vi "simple acq - used for Insight.vi"() -> ()   [LabVIEW 2015]
uses:
  AlazarTech/ATS-VI/6.0.8/ATS_ctl/ATS_Async_Status.ctl
  AlazarTech/ATS-VI/6.0.8/ATS_ctl/ATS_Global.ctl
  AlazarTech/ATS-VI/6.0.8/ATS_ctl/Record.ctl
  AlazarTech/ATS-VI/6.0.8/ATS_ctl/Clock.ctl
  AlazarTech/ATS-VI/6.0.8/ATS_ctl/ClockSource.ctl
  AlazarTech/ATS-VI/6.0.8/ATS_ctl/ClockRate.ctl
  AlazarTech/ATS-VI/6.0.8/ATS_ctl/ClockEdge.ctl
  AlazarTech/ATS-VI/6.0.8/ATS_ctl/InputCtrl.ctl
  AlazarTech/ATS-VI/6.0.8/ATS_ctl/Coupling.ctl
  AlazarTech/ATS-VI/6.0.8/ATS_ctl/Range.ctl
  AlazarTech/ATS-VI/6.0.8/ATS_ctl/Impedance.ctl
  AlazarTech/ATS-VI/6.0.8/ATS_ctl/Bandwidth.ctl
  AlazarTech/ATS-VI/6.0.8/ATS_ctl/Trigger.ctl
  AlazarTech/ATS-VI/6.0.8/ATS_ctl/TriggerOperation.ctl
  AlazarTech/ATS-VI/6.0.8/ATS_ctl/TriggerEngine.ctl
  AlazarTech/ATS-VI/6.0.8/ATS_ctl/ExtTrigger.ctl
  AlazarTech/ATS-VI/6.0.8/ATS_ctl/ExtTrigRange.ctl
  AlazarTech/ATS-VI/6.0.8/ATS_ctl/ATS_Async_Ctrl.ctl
  AlazarTech/ATS-VI/6.0.8/ATS_ctl/ATS_Async_Mode.ctl
  AlazarTech/ATS-VI/6.0.8/ATS_ctl/ATS_Async_Setting.ctl
  AlazarTech/ATS-VI/6.0.8/ATS_ctl/ATS_DMA_Channel.ctl
  AlazarTech/ATS-VI/6.0.8/ATS_ctl/ATS_ReadSamples.ctl
  AlazarTech/ATS-VI/6.0.8/ATS_ctl/Device_Ctrl.ctl
  <vilib>/Utility/file.llb/Read From Spreadsheet File (DBL).vi
panel:
  in  "saving":bool
  out "Record.Length":u32
  out "offset":i16
  out "mult":dbl
  in  "result":bool
  out "path":path
  in  "save sweep":bool
  in  "use DVV":bool=TRUE
  out "dvv":dbl[](array[numeric]) format="%0.3f"
  in  "file path (dialog if empty)":path=path "\\\\192.168.1.100\\data/DVV.txt"
  in  "Setup_In":T1={"Record"={"Count"=1, "Presize"=0, "Length"=2784}, "Clock"={"ClckSource"=enum."External", "ClckRate"=12, "ClckEdge"=0, "Decimation"=0}, "Input A"={"Coupling"=enum."DC", "Range"=5, "Impedance"=enum."50 ohms", "Bandwidth"=enum."Full Bandwidth"}, "Input B"={"Coupling"=enum."DC", "Range"=6, "Impedance"=enum."50 ohms", "Bandwidth"=enum."Full Bandwidth"}, "Trigger"={"TrigOperation"=enum."Only X", "Timeout (s)"=1.0, "Trig. Delay"=0, "Engine X"={"Source"=enum."External", "Slope"=enum."Positive", "Level"=150}, "Engine Y"={"Source"=enum."Disable", "Slope"=enum."Positive", "Level"=128}, "ExtTrigControl"={"Coupling"=enum."DC", "Range"=enum."TTL"}}} {"Clock"."ClckEdge" items=["Rising", "Falling"]; "Clock"."ClckRate" items=["1 kS/s", "2 kS/s", "5 kS/s", "10 kS/s", "20 kS/s", "50 kS/s", "100 kS/s", "200 kS/s", "500 kS/s", "1 MS/s", "2 MS/s", "5 MS/s", "10 MS/s", "20 MS/s", "50 MS/s", "100 MS/s", "250 MS/s", "500 MS/s"]; "Input B"."Range" items=["40mV", "100mV", "200mV", "400mV", "1 V", "2 V", "4 V"]; "Trigger"."Timeout (s)" format="%.2f"; "Input A"."Range" items=["40mV", "100mV", "200mV", "400mV", "1 V", "2 V", "4 V"]}
  out "Async_Status":T17
  out "error out":errorcluster
  out "Waveform Graph":dbl[](graph)
  in  "Stop Button":bool
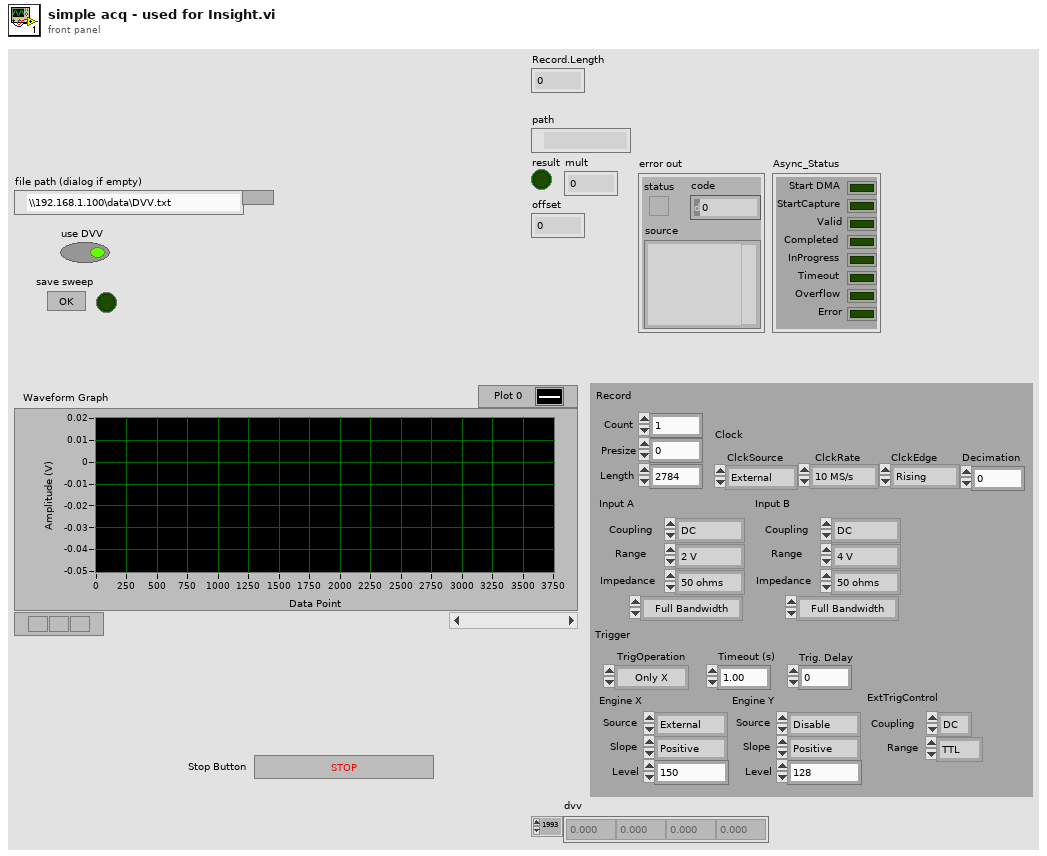
[diagram p1: front panel]
types:
  T1 = typedef "ATS_Global.ctl" = cluster{"Record":T2, "Clock":T3, "Input A":T7, "Input B":T7, "Trigger":T12}
  T2 = typedef "Record.ctl" = cluster{"Count":u32, "Presize":u32, "Length":u32}
  T3 = typedef "Clock.ctl" = cluster{"ClckSource":T4, "ClckRate":T5, "ClckEdge":T6, "Decimation":u32}
  T4 = typedef "ClockSource.ctl" = enum16{"Internal", "External", "Medium Ext.", "Slow Ext.", "Ext. AC", "Ext. DC", "Ext. (PLL)"}
  T5 = typedef "ClockRate.ctl" = u32
  T6 = typedef "ClockEdge.ctl" = u16
  T7 = typedef "InputCtrl.ctl" = cluster{"Coupling":T8, "Range":T9, "Impedance":T10, "Bandwidth":T11}
  T8 = typedef "Coupling.ctl" = enum16{"AC", "DC"}
  T9 = typedef "Range.ctl" = u32
  T10 = typedef "Impedance.ctl" = enum16{"1M ohms", "50 ohms"}
  T11 = typedef "Bandwidth.ctl" = enum16{"Full Bandwidth", "Reduce Bandwidth"}
  T12 = typedef "Trigger.ctl" = cluster{"TrigOperation":T13, "Timeout (s)":dbl, "Trig. Delay":u32, "Engine X":T14, "Engine Y":T14, "ExtTrigControl":T15}
  T13 = typedef "TriggerOperation.ctl" = enum16{"Only X", "Only Y", "X or Y", "X and Y", "X xor Y", "X and not Y", "not X and Y"}
  T14 = typedef "TriggerEngine.ctl" = cluster{"Source":enum32{"Chan_A", "Chan_B", "External", "Disable"}, "Slope":enum32{"Positive", "Negative"}, "Level":u32}
  T15 = typedef "ExtTrigger.ctl" = cluster{"Coupling":T8, "Range":T16}
  T16 = typedef "ExtTrigRange.ctl" = enum16{"1 V", "5 V", "TTL"}
  T17 = typedef "ATS_Async_Status.ctl" = cluster{"Start DMA":bool, "StartCapture":bool, "Valid":bool, "Completed":bool, "InProgress":bool, "Timeout":bool, "Overflow":bool, "Error":bool}
  T18 = typedef "ATS_ReadSamples.ctl" = cluster{"Offset":i32, "Length":u32}
  T19 = typedef "ATS_DMA_Channel.ctl" = enum16{"Channel_A", "Channel_B", "A & B"}
  T20 = typedef "ATS_Async_Setting.ctl" = cluster{"UseHeader":u32, "Rec/Buffer":u32, "Total_Rec":u32, "DataBuffer":bool, "GetProcessedData":bool}
  T21 = typedef "ATS_Async_Mode.ctl" = enum16{"Continuous", "Triggered", "No-Pre-Trigger", "Traditional"}
  T22 = typedef "ATS_Async_Ctrl.ctl" = enum16{"SetupDMA", "StartCapture", "Get", "Get_Stream", "Abort", "Stop"}
  T23 = typedef "Device_Ctrl.ctl" = enum16{"Status", "About", "Arm", "ForceTrig", "Abort", "Initialize", "Init (NoPreset)", "Info", "Close", "Calibrate", "SetManually", "LED_ON", "LED_OFF"}
  T24 = enum16{"open", "replace", "create", "open or create", "replace or create", "replace or create with confirmation"}
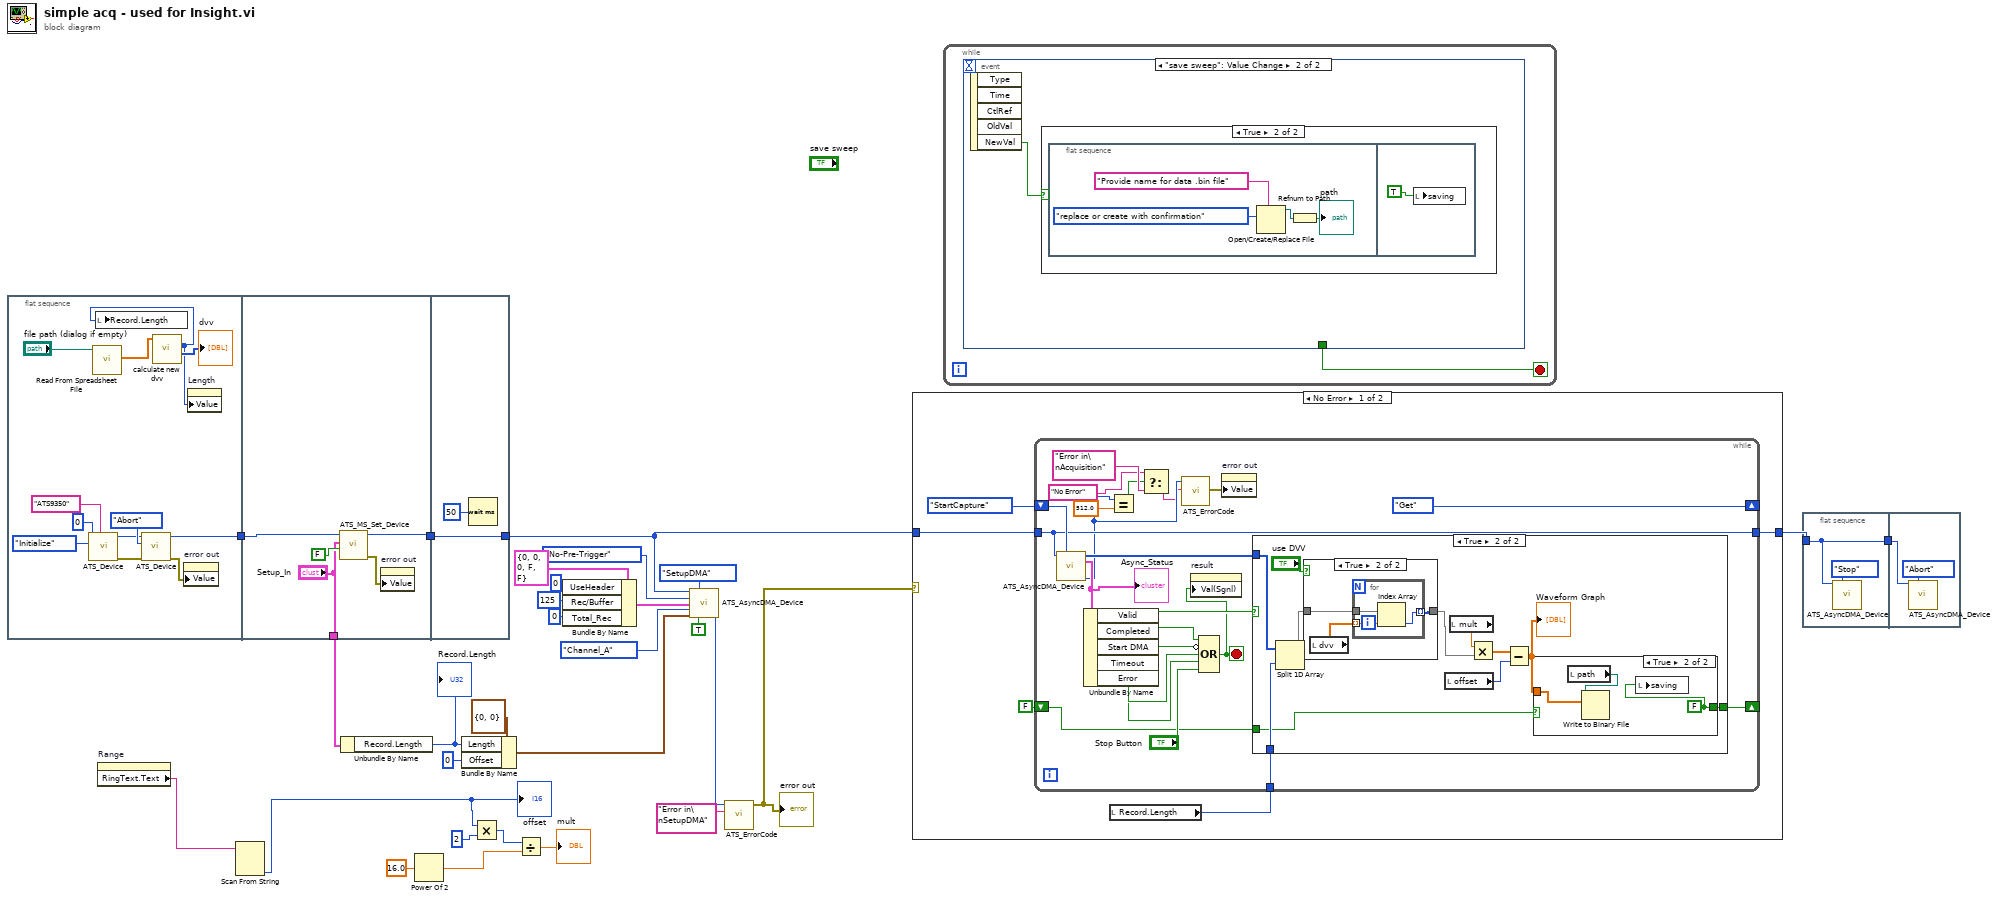
[diagram p0: block diagram]
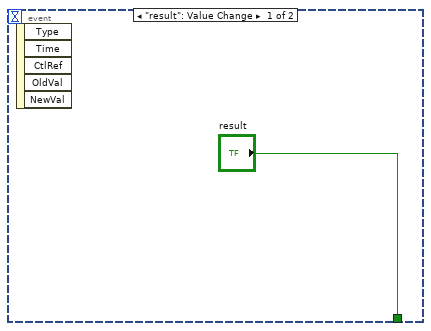
[diagram p2: hidden frame]
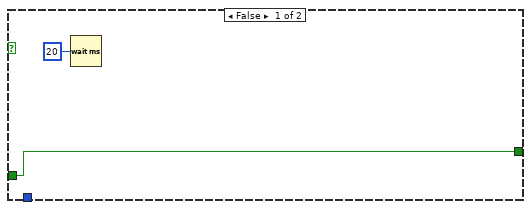
[diagram p4: hidden frame]
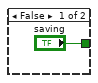
[diagram p5: hidden frame]
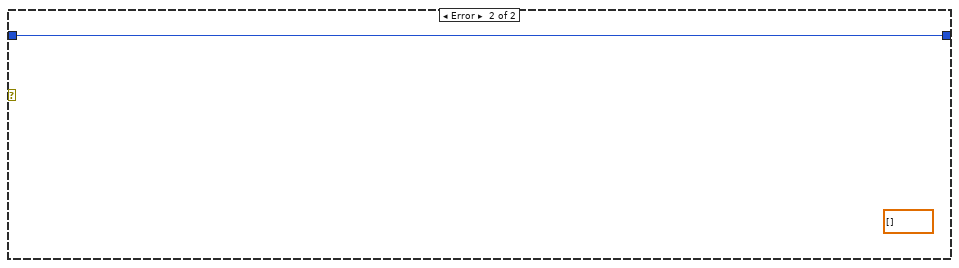
[diagram p7: hidden frame]
diagram:
  n1 = flat-sequence {
    tunnel: [w35] -> w26
    tunnel: w26 -> [w46]
    tunnel: [w45] -> w25
    tunnel: ["Setup_In"] -> w8
    tunnel: [w47] -> w27
    tunnel: w25 -> [w47]
    frame #0 {
      n2 = call "ATS_Device.vi"("BoardToVerify"="ATS9350", "DevCtrl"=Device_Ctrl."Initialize", "DeviceIn"=0 ("Device")) -> ("error out"=w40:errorcluster, "DeviceOut"=w36:i32)  [unwired: 2 in, 5 out]
      n3 = call-poly <vilib>:"Read From Spreadsheet File.vi"("file path (dialog if empty)"="file path (dialog if empty)") -> ("first row"=w32:dbl[])  [unwired: 6 in, 4 out]
      n4 = call "ATS_Device.vi"("error in (no error)"=w40, "DevCtrl"=Device_Ctrl."Abort", "DeviceIn"=w36) -> ("error out"=w34:errorcluster, "DeviceOut"=w35:i32)  [unwired: 2 in, 5 out]
      n5 = call "calculate new dvv.vi"("dvv"=w32) -> ("DVV*"=→"dvv":u32[], "Record Points"=w30:i32)  [unwired: 9 in]
      n6 = local write "Record.Length"(w30) -> ()
      n7 = property on="error out" class="Clust (strict)"("Value"=w34) -> ()  [unwired: 2 in, 2 out]
      n8 = property on="Length" class="DigNum (strict)"("Value"=w30) -> ()  [unwired: 2 in, 2 out]
    }
    frame #1 {
      n9 = call "ATS_MS_Set_Device.vi"("Set_Manually (F)"=FALSE, "Setup_In"="Setup_In", "DeviceIn"=w46) -> ("error out"=w43:errorcluster, "DeviceOut"=w45:i32)  [unwired: 3 in, 4 out]
      n10 = property on="error out" class="Clust (strict)"("Value"=w43) -> ()  [unwired: 2 in, 2 out]
    }
    frame #2 {
      n11 = Wait (ms)(milliseconds to wait=u32 50) -> ()  [unwired: 1 out]
    }
  }
  n12 = property on="Range" class="Ring (strict)"() -> ("RingText.Text"=w2:string)  [unwired: 2 in, 2 out]
  n13 = Scan From String(input string=w2) -> (output 1=w1:i16)  [unwired: 4 in, 3 out]
  "offset" <- w1
  n14 = Unbundle By Name(w8) -> ("Record.Length"=w14:u32)
  "Record.Length" <- w14
  n15 = Power Of 2(x=16.0) -> (2^x=w6:dbl)
  n16 = Bundle By Name(cluster=T18 {"Offset"=0, "Length"=0} ("ReadSamples"), "Length"=w14, "Offset"=0) -> (w16:T18)
  n17 = Multiply(x=w1, y=2 ("Offset")) -> (x*y=w4:i32)
  n18 = Divide(x=w4, y=w6) -> (x/y=→"mult":dbl)
  n19 = Bundle By Name(cluster=T20 {"UseHeader"=0, "Rec/Buffer"=0, "Total_Rec"=0, "DataBuffer"=FALSE, "GetProcessedData"=FALSE} ("Async_Setting"), "UseHeader"=u32 0, "Rec/Buffer"=u32 125, "Total_Rec"=u32 0) -> (w21:T20)
  n20 = call "ATS_AsyncDMA_Device.vi"("DeviceIn"=w27, "ATS_Async_Ctrl"=ATS_Async_Ctrl."SetupDMA" ("ATS_DMA_Ctrl"), "Async_Mode"=ATS_Async_Mode."No-Pre-Trigger", "Async_Setting"=w21, "Channel"=ATS_DMA_Channel."Channel_A", "ReadSamples"=w16, "Start Now / Wait"=TRUE) -> ("Return Code"=w13:u32)  [unwired: 4 in, 4 out]
  n21 = call "ATS_ErrorCode.vi"("Message"="Error in\nSetupDMA", "ErrorCode"=w13) -> ("error out"=w12:errorcluster)  [unwired: 5 in]
  "error out" <- w12
  n22 = case shown="No Error" w12 {
    tunnel: w27 -> [w53 w100]
    tunnel: [w51 w100] -> w10
    frame No Error {
      n23 = local read "Record.Length"() -> (w50:u32)
      n24 = while {
        tunnel: w53 -> [w66]
        shift-right: [ATS_Async_Ctrl."Get" ("ATS_Async_Ctrl")] -> _
        shift-left: ATS_Async_Ctrl."StartCapture" ("ATS_Async_Ctrl") -> [w71]
        tunnel: [w66] -> w51
        tunnel: w50 -> [w62]
        shift-right: [w61] -> _
        shift-left: FALSE ("Boolean") -> [w60]
        stop <- w63 stop-if-true
        n25 = call "ATS_AsyncDMA_Device.vi"("DeviceIn"=w66, "ATS_Async_Ctrl"=w71) -> ("Buffer"=w64:u16[], "Async_Status"=w67:T17, "Return Code"=w55:u32)  [unwired: 9 in, 2 out]
        "Async_Status" <- w67
        n26 = Unbundle By Name(w67) -> ("Valid"=w69:bool, "Completed"=w73:bool, "Start DMA"=w74:bool, "Timeout"=w75:bool, "Error"=w72:bool)
        n27 = Equal?(x=w55, y=512.0) -> (x = y?=w57:bool)
        n28 = Select(t="No Error" ("Message"), s=w57, f="Error in\nAcquisition" ("Message")) -> (s? t:f=w54:string)
        n29 = call "ATS_ErrorCode.vi"("Message"=w54, "ErrorCode"=w55) -> ("error out"=w65:errorcluster)  [unwired: 5 in]
        n30 = Compound Arithmetic op=OR(w73, invert w74, w75, w72, "Stop Button") -> (w63:bool)
        n31 = property on="result" class="Bool (strict)"("Val(Sgnl)"=w63) -> ()  [unwired: 2 in, 2 out]
        n32 = property on="error out" class="Clust (strict)"("Value"=w65) -> ()  [unwired: 2 in, 2 out]
        n33 = case shown="True" w69 {
          tunnel: w64 -> [_ w82]
          tunnel: w62 -> [_ w80]
          tunnel: [w76 w79] -> w61
          tunnel: w60 -> [w76 w78]
          frame False {
            n34 = Wait (ms)(milliseconds to wait=u32 20) -> ()  [unwired: 1 out]
          }
          frame True {
            n35 = Split 1D Array(array=w82, index=w80) -> (first subarray=w81:u16[])  [unwired: 1 out]
            n36 = case shown="True" "use DVV" {
              tunnel: w81 -> [w93 w96]
              tunnel: [w93 w94] -> w84
              frame False {
              }
              frame True {
                n37 = local read "dvv"() -> (w95:dbl[])
                n38 = for {
                  tunnel: w96 -> [w97]
                  tunnel: [w99] -> w94 mode=indexing
                  tunnel: w95 -> [w98] mode=indexing
                  n39 = Index Array(array=w97, index=w98) -> (element=w99:u16)
                }
              }
            }
            n40 = local read "offset"() -> (w86:i16)
            n41 = local read "mult"() -> (w85:dbl)
            n42 = Multiply(x=w85, y=w84) -> (x*y=w87:dbl[])
            n43 = Subtract(x=w87, y=w86) -> (x-y=w83:dbl[])
            "Waveform Graph" <- w83
            n44 = case shown="True" w78 {
              tunnel: w83 -> [_ w91]
              tunnel: ["saving" w90] -> w79
              frame False {
              }
              frame True {
                w90 = FALSE ("Boolean")
                n45 = local read "path"() -> (w92:path)
                n46 = Write to Binary File(file (use dialog)=w92, data=w91) -> ()  [unwired: 4 in, 3 out]
                n47 = local write "saving"(w90) -> ()
              }
            }
          }
        }
      }
    }
    frame Error {
      (unwired) dbl[] []
    }
  }
  n48 = while {
    stop <- w101 stop-if-true
    n49 = event shown="[1] \"save sweep\": Value Change" {
      selector: _ -> [_ _]
      dyn-events: _ -> [_ _]
      timeout: _ -> [_ _]
      tunnel: ["result" _] -> w101
      event "result": Value Change {
        n50 = event-data() -> ()  [unwired: 1 in, 5 out]
      }
      event "save sweep": Value Change {
        n51 = event-data() -> ("NewVal"=w103:bool)  [unwired: 1 in, 4 out]
        n52 = case shown="True" w103 {
          frame False {
          }
          frame True {
            n53 = flat-sequence {
              frame #0 {
                n54 = Open/Create/Replace File(prompt="Provide name for data .bin file", operation (0:open)=T24."replace or create with confirmation") -> (refnum out=w105:refnum<file>)  [unwired: 4 in, 2 out]
                n55 = Refnum to Path(1:w105) -> (0:→"path":path)
              }
              frame #1 {
                n56 = local write "saving"(TRUE) -> ()
              }
            }
          }
        }
      }
    }
  }
  n57 = flat-sequence {
    tunnel: w10 -> [w109]
    tunnel: [w109] -> w11
    tunnel: w11 -> [w111]
    frame #0 {
      n58 = call "ATS_AsyncDMA_Device.vi"("DeviceIn"=w109, "ATS_Async_Ctrl"=ATS_Async_Ctrl."Stop" ("ATS_DMA_Ctrl")) -> ()  [unwired: 9 in, 5 out]
    }
    frame #1 {
      n59 = call "ATS_AsyncDMA_Device.vi"("DeviceIn"=w111, "ATS_Async_Ctrl"=ATS_Async_Ctrl."Abort" ("ATS_DMA_Ctrl")) -> ()  [unwired: 9 in, 5 out]
    }
  }
